vi "Blynk Login.vi"(7 "Auth Token":string, 8 "error in (no error)":errorcluster, 10 "port (8442)":u16, 11 "address (cloud.blynk.cc)":string) -> (0 "error out":errorcluster, 2 "STATUS":u16, 3 "connection out":refnum<k5>)   [LabVIEW 2014]
uses:
  utilities/MsgType.ctl
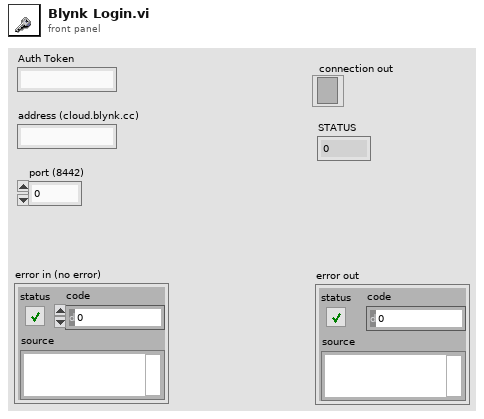
[diagram p1: front panel]
types:
  T1 = typedef "MsgType.ctl" = enum8{"RSP", "REGISTER", "LOGIN", "SAVE_PROF", "LOAD_PROF", "GET_TOKEN", "PING", "ACTIVATE", "DEACTIVATE", "REFRESH", "UNDEFINED0", "UNDEFINED1", "TWEET", "EMAIL", "NOTIFY", "BRIDGE", "UNDEFINED2", "UNDEFINED3", "UNDEFINED4", "UNDEFINED5", "HW"}
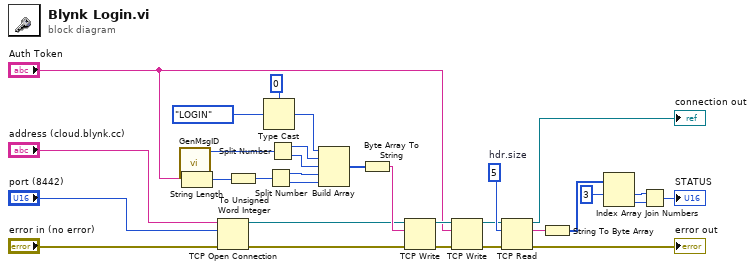
[diagram p0: block diagram]
diagram:
  w18 = 5  # hdr.size
  n1 = call "GenMsgID.vi"() -> ("MsgID"=w22:u16)  [unwired: 10 in, 1 out]
  n2 = String Length(string="Auth Token") -> (length=w11:i32)
  n3 = TCP Open Connection(address="address (cloud.blynk.cc)", remote port or service name="port (8442)", error in (no error)="error in (no error)") -> (connection ID=w4:refnum<k5>, error out=w5:errorcluster)  [unwired: 2 in]
  n4 = To Unsigned Word Integer(number=w11) -> (unsigned 16bit integer=w13:u16)
  n5 = Type Cast(type=u8 0, x=MsgType."LOGIN") -> (*(type *) &x=w24:u8)
  n6 = Split Number(x=w13) -> (hi(x)=w14:u8, lo(x)=w15:u8)
  n7 = Split Number(x=w22) -> (hi(x)=w21:u8, lo(x)=w12:u8)
  n8 = Build Array(w24, w21, w12, w14, w15) -> (w16:u8[])
  n9 = Byte Array To String(unsigned byte array=w16) -> (string=w17:string)
  n10 = TCP Write(connection ID=w4, data in=w17, error in (no error)=w5) -> (connection ID out=w9:refnum<k5>, error out=w10:errorcluster)  [unwired: 1 in, 1 out]
  n11 = TCP Write(connection ID=w9, data in="Auth Token", error in (no error)=w10) -> (connection ID out=w7:refnum<k5>, error out=w8:errorcluster)  [unwired: 1 in, 1 out]
  n12 = TCP Read(connection ID=w7, bytes to read=w18, error in (no error)=w8) -> (connection ID out=→"connection out":refnum<k5>, data out=w19:string, error out=→"error out":errorcluster)  [unwired: 2 in]
  n13 = String To Byte Array(string=w19) -> (unsigned byte array=w20:u8[])
  n14 = Index Array(array=w20, index #1=3 ("index")) -> (element #1=w27:u8, element #2=w28:u8)  [unwired: 1 in]
  n15 = Join Numbers(hi=w27, lo=w28) -> ((hi.lo)=→"STATUS":u16)
